vi "sslSimulationProtocolMoveLocalVelocity.vi"(8 "error in (no error)":errorcluster, 10 "robot":T1, 11 "Communication in":refnum<class "Communication.lvclass">) -> (0 "error out":errorcluster, 2 "MoveLocalVelocity":u8[](array[numeric]), 3 "Communication out":refnum<class "Communication.lvclass">)   [LabVIEW 2020, in "Communication.lvclass"]
uses:
  Communication.lvclass
  Convert AI Robot to Robot Command Folder/grSim/grSim Robot Command.ctl
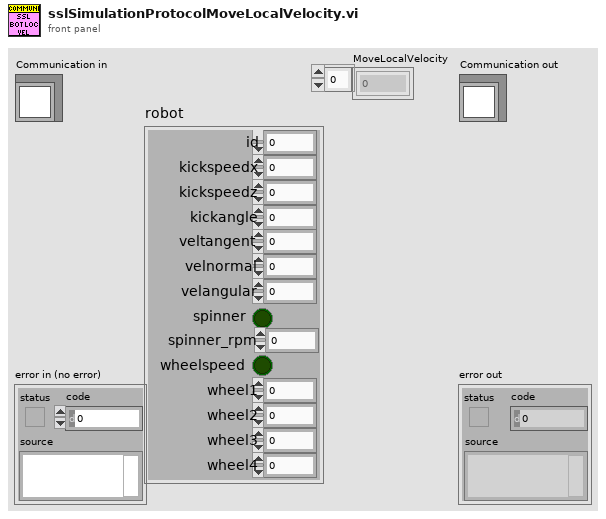
[diagram p1: front panel]
types:
  T1 = typedef "grSim Robot Command.ctl" = cluster{"id":u32, "kickspeedx":sgl, "kickspeedz":sgl, "veltangent":sgl, "velnormal":sgl, "velangular":sgl, "spinner":bool, "wheelspeed":bool, "wheel1":sgl, "wheel2":sgl, "wheel3":sgl, "wheel4":sgl, "kickangle":sgl, "spinner_rpm":sgl}
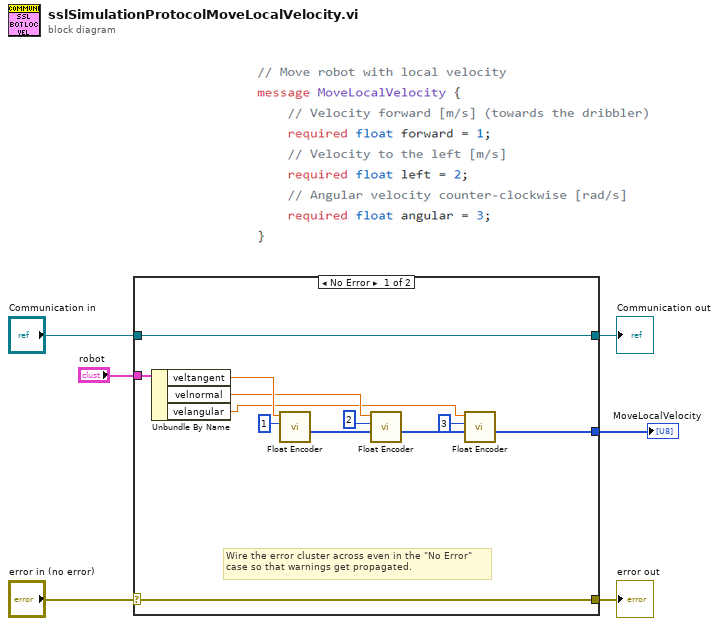
[diagram p0: block diagram]
diagram:
  n1 = case shown="No Error" "error in (no error)" {
    selector: "error in (no error)" -> [w17 w20]
    tunnel: [w17 w20] -> w5
    tunnel: [w18 w19] -> w3
    tunnel: "Communication in" -> [w18 w19]
    tunnel: [w11 _] -> w2
    tunnel: "robot" -> [w10 _]
    frame No Error {
      # "Wire the error cluster across even in the \"No Error\"\ncase so that warnings get propagated."
      n2 = Unbundle By Name(w10) -> ("veltangent"=w9:sgl, "velnormal"=w8:sgl, "velangular"=w7:sgl)
      n3 = call "Float Encoder.vi"("Key"=u32 1, "Value"=w9) -> ("Array"=w15:u8[])  [unwired: 9 in]
      n4 = call "Float Encoder.vi"("Array In"=w15, "Key"=u32 2, "Value"=w8) -> ("Array"=w13:u8[])  [unwired: 8 in]
      n5 = call "Float Encoder.vi"("Array In"=w13, "Key"=u32 3, "Value"=w7) -> ("Array"=w11:u8[])  [unwired: 8 in]
    }
    frame Error {
    }
  }
  "error out" <- w5
  "Communication out" <- w3
  "MoveLocalVelocity" <- w2
